vi "Add or Replace Element.vi"(8 "error in":errorcluster, 11 "XML Document in":refnum<class "XML Document.lvclass">) -> (0 "error out":errorcluster, 3 "XML Document out":refnum<class "XML Document.lvclass">)   [LabVIEW 2014, in "XML Document.lvclass"]
uses:
  XML Document.lvclass
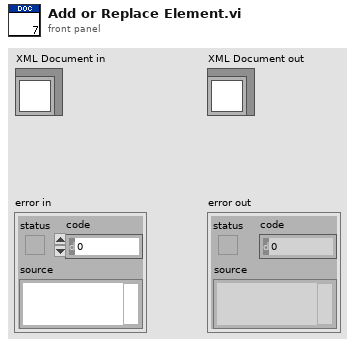
[diagram p1: front panel]
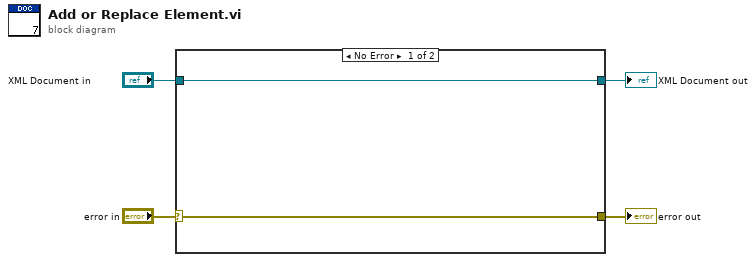
[diagram p0: block diagram]
diagram:
  n1 = case shown="No Error" "error in" {
    selector: "error in" -> [w5 w8]
    tunnel: [w5 w8] -> w3
    tunnel: [w6 w7] -> w1
    tunnel: "XML Document in" -> [w6 w7]
    frame No Error {
    }
    frame Error {
    }
  }
  "error out" <- w3
  "XML Document out" <- w1
